vi "LJLogUD.vi"() -> ()   [LabVIEW 2020]
panel:
  in  "Save Current Config":bool
  out "Device Config File Name":string
  out "Actual Interval (ms)":i32
  in  "Graphing parameters":T1(tab)
  in  "Graph?":bool[](array[boolean])
  out "Scaled":dbl[](array[numeric]) format="%.6f"
  in  "Scaling Equation":string[](array[string])=["y=a", "y=b", "y=c", "y=d", "y=e", "y=f", "y=g", "y=h", "y=i", "y=j", "y=k", "y=l", "y=m", "y=n", "y=o", "y=p"]
  out "Voltage":dbl[](array[numeric]) format="%.6f"
  in  "Ranges":u16[](array[ring])=[0, 0, 0, 0, 0, 0, 0, 0, 0, 0, 0, 0, 0, 0, 0, 0] items=["LJ_rgBIP10V", "LJ_rgBIP5V", "LJ_rgUNI5V", "LJ_rgUNI2P5V", "LJ_rgUNI1P25V", "LJ_rgBIP1V", "LJ_rgUNIP625V", "LJ_rgBIPP1V", "LJ_rgBIPP01V"]
  in  "-Ch":string[](array[string])=["199", "199", "199", "199", "199", "199", "199", "199", "199", "199", "199", "199", "199", "199", "199", "199"]
  in  "+Ch":string[](array[string])=["1", "2", "3", "4", "5", "6", "7", "8", "9", "10", "11", "12", "13", "14", "15", "16"]
  out "Scaled 2":dbl[](array[numeric]) format="%.6f"
  in  "Graph? 2":bool[](array[boolean])
  in  "Ranges 2":u16[](array[ring])=[0, 0, 0, 0, 0, 0, 0, 0, 0, 0, 0, 0, 0, 0, 0, 0] items=["LJ_rgBIP10V", "LJ_rgBIP5V", "LJ_rgUNI5V", "LJ_rgUNI2P5V", "LJ_rgUNI1P25V", "LJ_rgBIP1V", "LJ_rgUNIP625V", "LJ_rgBIPP1V", "LJ_rgBIPP01V"]
  in  "Scaling Equation 2":string[](array[string])=["y=a2", "y=b2", "y=c2", "y=d2", "y=e2", "y=f2", "y=g2", "y=h2", "y=i2", "y=j2", "y=k2", "y=l2", "y=m2", "y=n2", "y=o2", "y=p2"]
  out "Voltage 2":dbl[](array[numeric]) format="%.6f"
  in  "-Ch 2":string[](array[string])=["199", "199", "199", "199", "199", "199", "199", "199", "199", "199", "199", "199", "199", "199", "199", "199"]
  in  "+Ch 2":string[](array[string])=["X3-AIN4", "X3-AIN5", "X3-AIN6", "X3-AIN7", "X3-AIN8", "X3-AIN9", "X3-AIN10", "X3-AIN11", "X3-AIN12", "X3-AIN13", "X3-DAC0", "X3-DAC1", "X3-FIO0", "X3-FIO1", "X3-FIO2", "X3-FIO3"]
  in  "Graph? 3":bool[](array[boolean])
  in  "Ranges 3":u16[](array[ring])=[0, 0, 0, 0, 0, 0, 0, 0, 0, 0, 0, 0, 0, 0, 0, 0] items=["LJ_rgBIP10V", "LJ_rgBIP5V", "LJ_rgUNI5V", "LJ_rgUNI2P5V", "LJ_rgUNI1P25V", "LJ_rgBIP1V", "LJ_rgUNIP625V", "LJ_rgBIPP1V", "LJ_rgBIPP01V"]
  out "Scaled 3":dbl[](array[numeric]) format="%.6f"
  in  "Scaling Equation 3":string[](array[string])=["y=a3", "y=b3", "y=c3", "y=d3", "y=e3", "y=f3", "y=g3", "y=h3", "y=i3", "y=j3", "y=k3", "y=l3", "y=m3", "y=n3", "y=o3", "y=p3"]
  out "Voltage 3":dbl[](array[numeric]) format="%.6f"
  in  "-Ch 3":string[](array[string])=["199", "199", "199", "199", "199", "199", "199", "199", "199", "199", "199", "199", "199", "199", "199", "199"]
  in  "+Ch 3":string[](array[string])=["X3-FIO4", "X3-FIO5", "X3-FIO6", "X3-FIO7", "X4-AIN0", "X4-AIN1", "X4-AIN2", "X4-AIN3", "X4-AIN4", "X4-AIN5", "X4-AIN6", "X4-AIN7", "X4-AIN8", "X4-AIN9", "X4-AIN10", "X4-AIN11"]
  in  "Graph? 4":bool[](array[boolean])
  in  "Ranges 4":u16[](array[ring])=[0, 0, 0, 0, 0, 0, 0, 0, 0, 0, 0, 0, 0, 0, 0, 0] items=["LJ_rgBIP10V", "LJ_rgBIP5V", "LJ_rgUNI5V", "LJ_rgUNI2P5V", "LJ_rgUNI1P25V", "LJ_rgBIP1V", "LJ_rgUNIP625V", "LJ_rgBIPP1V", "LJ_rgBIPP01V"]
  out "Scaled 4":dbl[](array[numeric]) format="%.6f"
  in  "Scaling Equation 4":string[](array[string])=["y=a4", "y=b4", "y=c4", "y=d4", "y=e4", "y=f4", "y=g4", "y=h4", "y=i4", "y=j4", "y=k4", "y=l4", "y=m4", "y=n4", "y=o4", "y=p4"]
  out "Voltage 4":dbl[](array[numeric]) format="%.6f"
  in  "-Ch 4":string[](array[string])=["199", "199", "199", "199", "199", "199", "199", "199", "199", "199", "199", "199", "199", "199", "199", "199"]
  in  "+Ch 4":string[](array[string])=["X4-AIN12", "X4-AIN13", "X4-DAC0", "X4-DAC1", "X4-FIO0", "X4-FIO1", "X4-FIO2", "X4-FIO3", "X4-FIO4", "X4-FIO5", "X4-FIO6", "X4-FIO7", "X5-AIN0", "X5-AIN1", "X5-AIN2", "X5-AIN3"]
  in  "Graph? 5":bool[](array[boolean])
  in  "Ranges 5":u16[](array[ring])=[0, 0, 0, 0, 0, 0, 0, 0, 0, 0, 0, 0, 0, 0, 0, 0] items=["LJ_rgBIP10V", "LJ_rgBIP5V", "LJ_rgUNI5V", "LJ_rgUNI2P5V", "LJ_rgUNI1P25V", "LJ_rgBIP1V", "LJ_rgUNIP625V", "LJ_rgBIPP1V", "LJ_rgBIPP01V"]
  out "Scaled 5":dbl[](array[numeric]) format="%.6f"
  in  "Scaling Equation 5":string[](array[string])=["y=a5", "y=b5", "y=c5", "y=d5", "y=e5", "y=f5", "y=g5", "y=h5", "y=i5", "y=j5", "y=k5", "y=l5", "y=m5", "y=n5", "y=o5", "y=p5"]
  out "Voltage 5":dbl[](array[numeric]) format="%.6f"
  in  "-Ch 5":string[](array[string])=["199", "199", "199", "199", "199", "199", "199", "199", "199", "199", "199", "199", "199", "199", "199", "199"]
  in  "+Ch 5":string[](array[string])=["X5-AIN4", "X5-AIN5", "X5-AIN6", "X5-AIN7", "X5-AIN8", "X5-AIN9", "X5-AIN10", "X5-AIN11", "X5-AIN12", "X5-AIN13", "X5-DAC0", "X5-DAC1", "X5-FIO0", "X5-FIO1", "X5-FIO2", "X5-FIO3"]
  in  "Graph? 6":bool[](array[boolean])
  in  "Ranges 6":u16[](array[ring])=[0, 0, 0, 0, 0, 0, 0, 0] items=["LJ_rgBIP10V", "LJ_rgBIP5V", "LJ_rgUNI5V", "LJ_rgUNI2P5V", "LJ_rgUNI1P25V", "LJ_rgBIP1V", "LJ_rgUNIP625V", "LJ_rgBIPP1V", "LJ_rgBIPP01V"]
  out "Scaled 6":dbl[](array[numeric]) format="%.6f"
  in  "Scaling Equation 6":string[](array[string])=["y=a6", "y=b6", "y=c6", "y=d6"]
  out "Voltage 6":dbl[](array[numeric]) format="%.6f"
  in  "-Ch 6":string[](array[string])=["199", "199", "199", "199"]
  in  "+Ch 6":string[](array[string])=["X5-FIO4", "X5-FIO5", "X5-FIO6", "X5-FIO7"]
  in  "Change Working Directory":bool
  in  "Max File Size (Bytes)":i32=1048576 min=1 max=2000000000
  out "Waveform Graph":cluster{dbl, dbl, dbl[][]}(graph)={0.0, 0.5, []}
  in  "# Scans On Graph":i32=1000 min=0
  out "Address":string
  out "Device Type":string
  in  "SettlingFactor":u8
  in  "Resolution":u8
  in  "exit":bool
  in  "# Channels":i32=4 min=1
  out "# Of Iterations":i32
  in  "Interval (ms)":u32=500
  out "Current Data File":path
  in  "Data File Prefix":string="data"
  in  "Write To File":bool
  out "Error Message":string="No Error"
  # "Page 1"
  # "Page 2"
  # "Page 3"
  # "Page 5"
  # "Page 6"
  # "Page 4"
  # "- \"a\" - \"p\" correspond to the raw Voltage value from \n  the 1st through 16th row of each page.\n- The scaled output value is \"y\".\n- If your equation has an error, the output will be\n   zero."
  # "0"
  # "1"
  # "2"
  # "3"
  # "4"
  # "5"
  # "6"
  # "7"
  # "8"
  # "9"
  # "10"
  # "11"
  # "12"
  # "13"
  # "14"
  # "15"
  # "+Ch"
  # "-Ch"
  # "Ranges"
  # "Voltage"
  # "Scaling Equation"
  # "Scaled"
  # "Graph?"
  # "16"
  # "17"
  # "18"
  # "19"
  # "20"
  # "21"
  # "22"
  # "23"
  # "24"
  # "25"
  # "26"
  # "27"
  # "28"
  # "29"
  # "30"
  # "31"
  # "+Ch"
  # "-Ch"
  # "Ranges"
  # "Voltage"
  # "Scaling Equation"
  # "Scaled"
  # "Graph?"
  # "32"
  # "33"
  # "34"
  # "35"
  # "36"
  # "37"
  # "38"
  # "39"
  # "40"
  # "41"
  # "42"
  # "43"
  # "44"
  # "45"
  # "46"
  # "47"
  # "+Ch"
  # "-Ch"
  # "Ranges"
  # "Voltage"
  # "Scaling Equation"
  # "Scaled"
  # "Graph?"
  # "48"
  # "49"
  # "50"
  # "51"
  # "52"
  # "53"
  # "54"
  # "55"
  # "56"
  # "57"
  # "58"
  # "59"
  # "60"
  # "61"
  # "62"
  # "63"
  # "+Ch"
  # "-Ch"
  # "Ranges"
  # "Voltage"
  # "Scaling Equation"
  # "Scaled"
  # "Graph?"
  # "64"
  # "65"
  # "66"
  # "67"
  # "68"
  # "69"
  # "70"
  # "71"
  # "72"
  # "73"
  # "74"
  # "75"
  # "76"
  # "77"
  # "78"
  # "79"
  # "+Ch"
  # "-Ch"
  # "Ranges"
  # "Voltage"
  # "Scaling Equation"
  # "Scaled"
  # "Graph?"
  # "80"
  # "81"
  # "82"
  # "83"
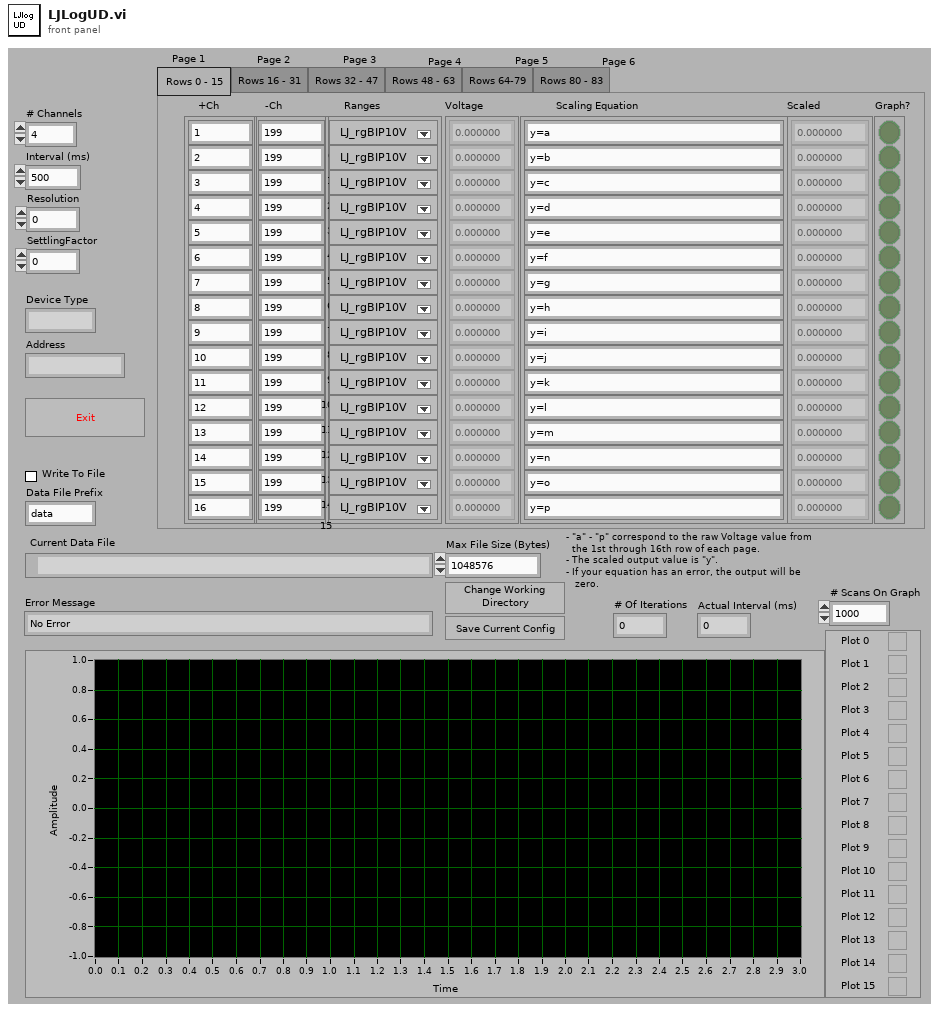
[diagram p1: front panel]
types:
  T1 = enum32{"Rows 0 - 15 ", "Rows 16 - 31", "Rows 32 - 47", "Rows 48 - 63", "Rows 64-79", "Rows 80 - 83"}
  T2 = cluster{"+Ch":string[], "-Ch":string[], "Ranges":u16[], "Scaling Equation":string[], "Graph?":bool[]}
  T3 = cluster{"# Channels":i32, "Channels Out":string[], "Channels Out":string[], u16[], string[]}
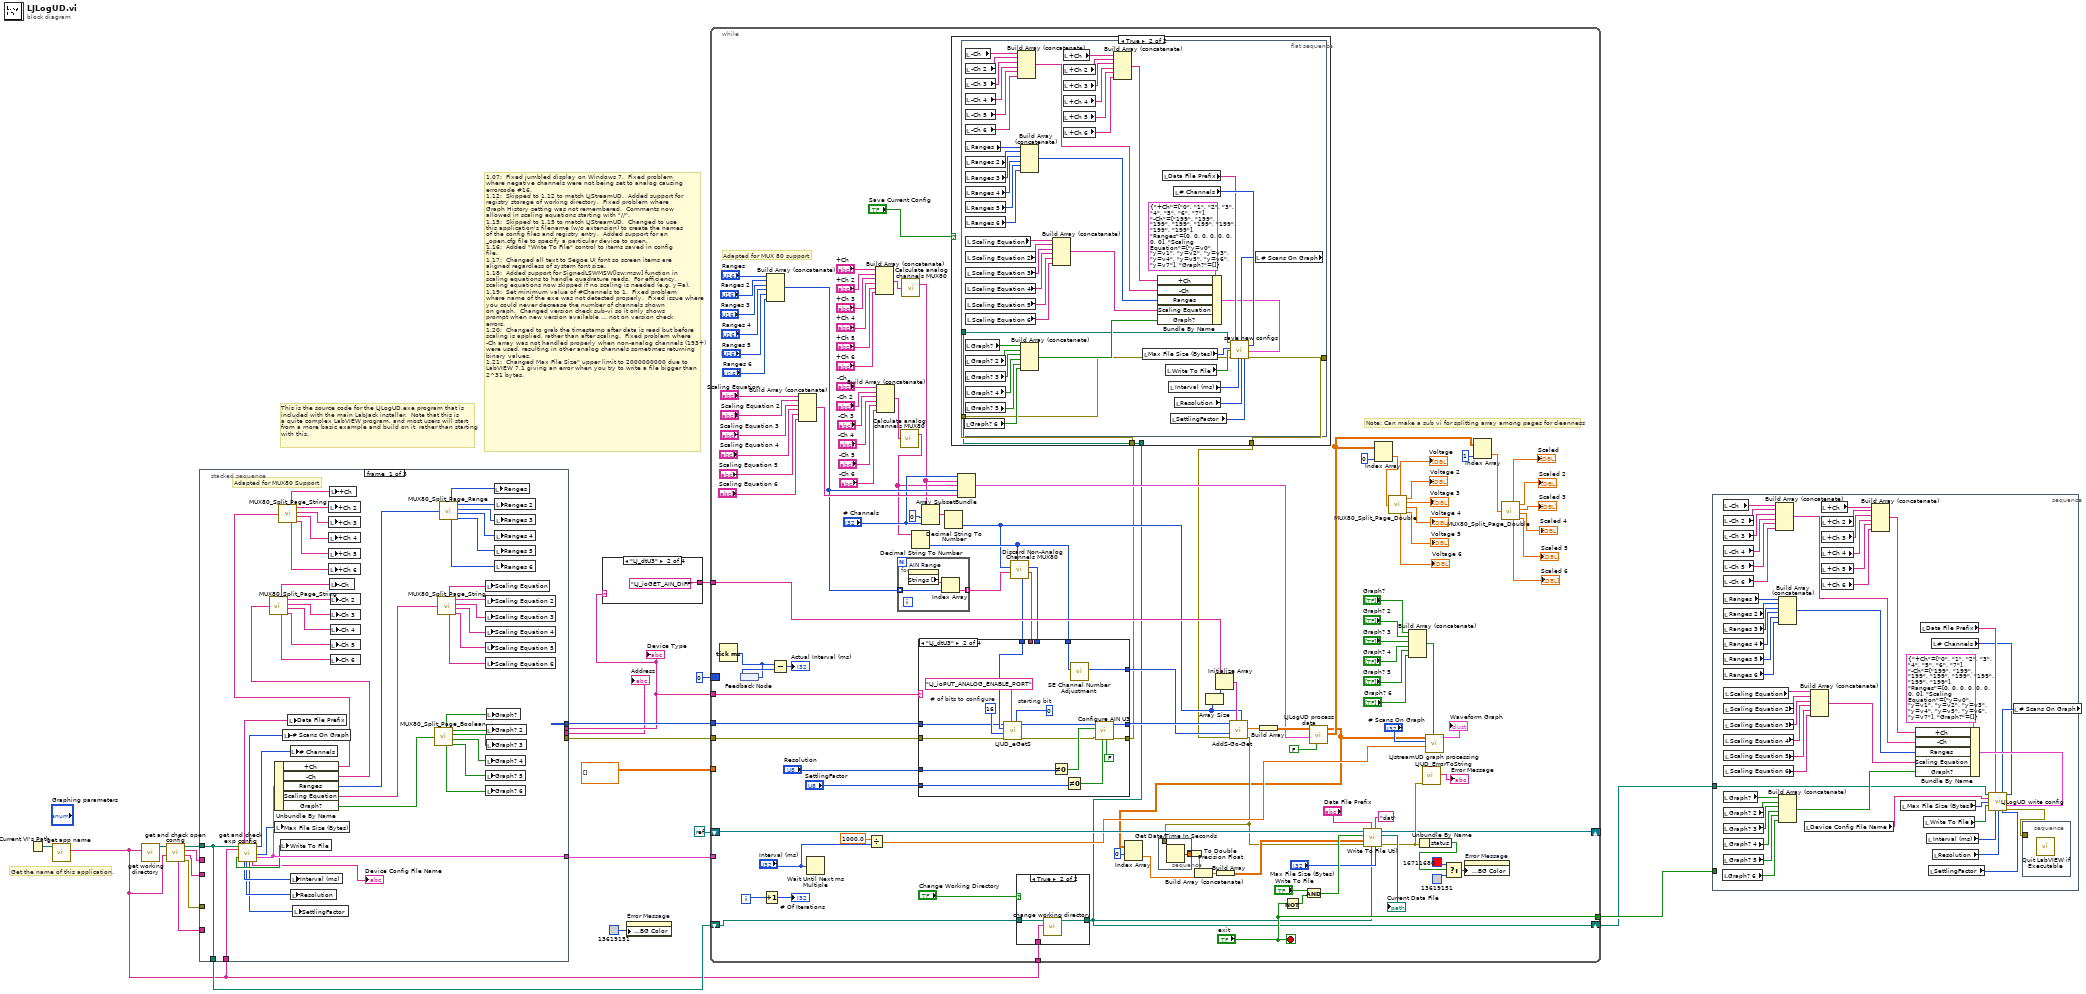
[diagram p0: block diagram]
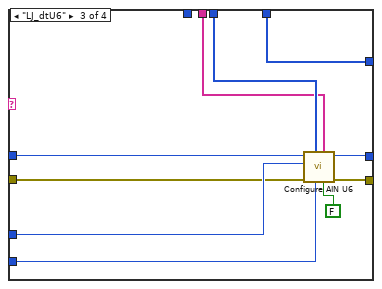
[diagram p5: hidden frame]
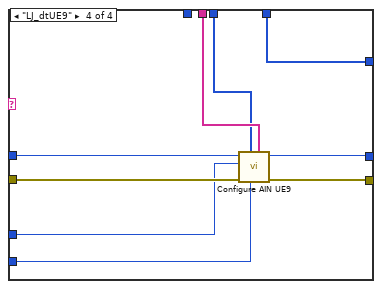
[diagram p6: hidden frame]
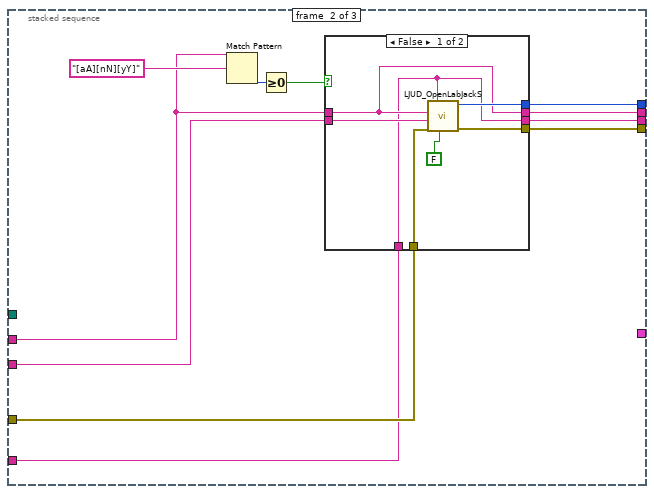
[diagram p7: hidden frame]
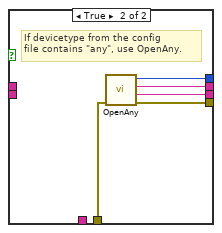
[diagram p8: hidden frame]
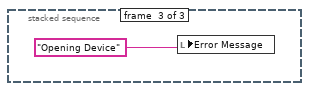
[diagram p9: hidden frame]
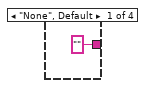
[diagram p10: hidden frame]
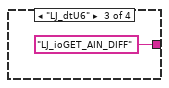
[diagram p11: hidden frame]
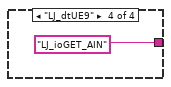
[diagram p12: hidden frame]
diagram:
  # "This is the source code for the LJLogUD.exe program that is\nincluded with the main LabJack installer.  Note that this is \na quite complex LabVIEW program, and most users will start\nfrom a more basic example and build on it, rather than starting\nwith this."
  # "Get the name of this application."
  # "1.07:  Fixed jumbled display on Windows 7.  Fixed problem\nwhere negative channels were not being set to analog causing\nerrorcode #16.\n1.12:  Skipped to 1.12 to match LJStreamUD.  Added support for\nregistry storage of working directory.  Fixed problem where\nGraph History setting was not remembered.  Comments now\nallowed in scaling equations starting with \"//\".\n1.15:  Skipped to 1.15 to match LJStreamUD.  Changed to use\nthis application's filename (w/o extension) to create the names\nof the config files and registry entry.  Added support for an\n_open.cfg file to specify a particular device to open.\n1.16:  Added \"Write To File\" control to items saved in config\nfile.\n1.17:  Changed all text to Segoe UI font so screen items are\naligned regardless of system font size.\n1.18:  Added support for SignedLSWMSW[lsw:msw] function in\nscaling equations to handle quadrature reads.  For efficiency,\nscaling equations now skipped if no scaling is needed (e.g. y=a).\n1.19:  Set minimum value of #Channels to 1.  Fixed problem\nwhere name of the exe was not detected properly.  Fixed issue where\nyou could never decrease the number of channels shown\non graph.  Changed version check sub-vi so it only shows\nprompt when new version available ... not on version check\nerrors.\n1.20:  Changed to grab the timestamp after data is read but before\nscaling is applied, rather than after scaling.  Fixed problem where\n-Ch array was not handled properly when non-analog channels (193+)\nwere used, resulting in other analog channels sometimes returning\nbinary values.\n1.21:  Changed Max File Size\" upper limit to 2000000000 due to\nLabVIEW 7.1 giving an error when you try to write a file bigger than\n2^31 bytes."
  n1 = Current VI's Path() -> (path=w10:path)
  n2 = call "get app name.vi"("Current VI's Path"=w10) -> ("App Name Without Extension"=w2:string)  [unwired: 4 in, 2 out]
  n3 = call "get working directory.vi"("Application Name"=w2) -> ("Working Directory"=w8:path)  [unwired: 9 in, 1 out]
  n4 = call "get and check open config.vi"("App Name"=w2, "Working Directory In"=w8) -> ("error out"=w6:errorcluster, "ConnectionType"=w4:string, "DeviceType"=w3:string, "Working Directory Out"=w7:path, "Identifier"=w5:string)  [unwired: 4 in, 1 out]
  n5 = stacked-sequence {
    tunnel: [w29 _ _] -> w18
    tunnel: [w26 _ _] -> w16
    tunnel: w2 -> [w33 _ _]
    tunnel: [_ w79 _] -> w14
    tunnel: [_ w78 _] -> w13
    tunnel: [_ w77 _] -> w12
    tunnel: [_ w76 _] -> w11
    tunnel: w7 -> [w26 _ _]
    tunnel: w6 -> [_ w72 _]
    tunnel: w5 -> [_ w71 _]
    tunnel: w4 -> [_ w70 _]
    tunnel: w3 -> [_ w69 _]
    frame #0 {
      # "Adapted for MUX80 Support"
      n6 = call "get and check exp config.vi"("Working Directory In"=w26, "App Name"=w33) -> ("Write To File"=w28:bool, "Data File Prefix"=w32:string, "Interval (ms)"=w27:u32, "Resolution"=w24:u8, "Graph History"=w31:i32, "SettlingFactor"=w23:u8, "Device Config File Name"=→"Device Config File Name":string, "# Channels"=w25:i32, "Max File Size (Bytes)"=w30:i32, "Channel Setup"=w29:T2)  [unwired: 6 in, 2 out]
      n7 = Unbundle By Name(w29) -> ("+Ch"=w56:string[], "-Ch"=w55:string[], "Ranges"=w47:u16[], "Scaling Equation"=w54:string[], "Graph?"=w40:bool[])
      n8 = call "MUX80_Split_Page_String.vi"("Array In"=w55) -> ("Page 1 out"=w62:string[], "Page 6 out"=w57:string[], "Page 2 out"=w61:string[], "Page 3 out"=w60:string[], "Page 4 out"=w59:string[], "Page 5 out"=w58:string[])
      n9 = local write "Max File Size (Bytes)"(w30) -> ()
      n10 = call "MUX80_Split_Page_String.vi"("Array In"=w56) -> ("Page 1 out"=w68:string[], "Page 6 out"=w63:string[], "Page 2 out"=w67:string[], "Page 3 out"=w66:string[], "Page 4 out"=w65:string[], "Page 5 out"=w64:string[])
      n11 = local write "Write To File"(w28) -> ()
      n12 = local write "# Scans On Graph"(w31) -> ()
      n13 = local write "Data File Prefix"(w32) -> ()
      n14 = local write "# Channels"(w25) -> ()
      n15 = local write "Interval (ms)"(w27) -> ()
      n16 = local write "Resolution"(w24) -> ()
      n17 = local write "SettlingFactor"(w23) -> ()
      n18 = local write "+Ch 2"(w67) -> ()
      n19 = local write "+Ch 3"(w66) -> ()
      n20 = local write "+Ch 4"(w65) -> ()
      n21 = local write "+Ch 5"(w64) -> ()
      n22 = local write "+Ch 6"(w63) -> ()
      n23 = local write "+Ch"(w68) -> ()
      n24 = local write "-Ch"(w62) -> ()
      n25 = local write "-Ch 2"(w61) -> ()
      n26 = local write "-Ch 3"(w60) -> ()
      n27 = local write "-Ch 4"(w59) -> ()
      n28 = local write "-Ch 5"(w58) -> ()
      n29 = local write "-Ch 6"(w57) -> ()
      n30 = call "MUX80_Split_Page_Boolean.vi"("Array In"=w40) -> ("Page 1 out"=w39:bool[], "Page 6 out"=w34:bool[], "Page 2 out"=w38:bool[], "Page 3 out"=w37:bool[], "Page 4 out"=w36:bool[], "Page 5 out"=w35:bool[])
      n31 = call "MUX80_Split_Page_String.vi"("Array In"=w54) -> ("Page 1 out"=w53:string[], "Page 6 out"=w48:string[], "Page 2 out"=w52:string[], "Page 3 out"=w51:string[], "Page 4 out"=w50:string[], "Page 5 out"=w49:string[])
      n32 = call "MUX80_Split_Page_Range.vi"("Array In"=w47) -> ("Page 1 out"=w46:u16[], "Page 6 out"=w41:u16[], "Page 2 out"=w45:u16[], "Page 3 out"=w44:u16[], "Page 4 out"=w43:u16[], "Page 5 out"=w42:u16[])
      n33 = local write "Scaling Equation"(w53) -> ()
      n34 = local write "Scaling Equation 2"(w52) -> ()
      n35 = local write "Scaling Equation 3"(w51) -> ()
      n36 = local write "Scaling Equation 4"(w50) -> ()
      n37 = local write "Scaling Equation 5"(w49) -> ()
      n38 = local write "Scaling Equation 6"(w48) -> ()
      n39 = local write "Graph? 4"(w36) -> ()
      n40 = local write "Graph? 5"(w35) -> ()
      n41 = local write "Graph? 6"(w34) -> ()
      n42 = local write "Graph?"(w39) -> ()
      n43 = local write "Graph? 2"(w38) -> ()
      n44 = local write "Graph? 3"(w37) -> ()
      n45 = local write "Ranges"(w46) -> ()
      n46 = local write "Ranges 2"(w45) -> ()
      n47 = local write "Ranges 3"(w44) -> ()
      n48 = local write "Ranges 4"(w43) -> ()
      n49 = local write "Ranges 5"(w42) -> ()
      n50 = local write "Ranges 6"(w41) -> ()
    }
    frame #1 {
      n51 = Match Pattern(string=w69, regular expression="[aA][nN][yY]") -> (offset past match=w75:i32)  [unwired: 1 in, 3 out]
      n52 = Greater Or Equal To 0?(x=w75) -> (x >= 0?=w73:bool)
      n53 = case shown="False" w73 {
        tunnel: [w86 w91] -> w79
        tunnel: [w82 w90] -> w78
        tunnel: [w80 w89] -> w77
        tunnel: [w85 w88] -> w76
        tunnel: w71 -> [w80 _]
        tunnel: w69 -> [w82 _]
        tunnel: w70 -> [w81 _]
        tunnel: w72 -> [w83 w87]
        frame False {
          n54 = call "LJUD_OpenLabJackS.vi"("FirstFound"=FALSE, "Address"=w80, "error in"=w83, "ConnectionType"=w81, "DeviceType"=w82) -> ("error out"=w85:errorcluster, "Handle"=w86:i32)  [unwired: 4 in, 1 out]
        }
        frame True {
          # "If devicetype from the config\nfile contains \"any\", use OpenAny."
          n55 = call "OpenAny.vi"("error in"=w87) -> ("error out"=w88:errorcluster, "Address Found"=w89:string, "Device Type Found"=w90:string, "Handle"=w91:i32)  [unwired: 7 in]
        }
      }
    }
    frame #2 {
      n56 = local write "Error Message"("Opening Device" ("Error Message")) -> ()
    }
  }
  "Device Type" <- w13
  "Address" <- w12
  n57 = case shown="\"LJ_dtU3\"" w13 {
    tunnel: ["" ("IOType") "LJ_ioGET_AIN_DIFF" ("IOType") "LJ_ioGET_AIN_DIFF" ("IOType") "LJ_ioGET_AIN" ("IOType")] -> w20
    frame "None", Default {
    }
    frame "LJ_dtU3" {
    }
    frame "LJ_dtU6" {
    }
    frame "LJ_dtUE9" {
    }
  }
  n58 = property on="Error Message" class="Str"("Text.Text Colors:BG Color"=u32 13619151) -> ()  [unwired: 2 in, 2 out]
  n59 = while {
    shift-left: w16 -> [w99]
    shift-right: [w98] -> w15
    tunnel: w2 -> [w170]
    tunnel: dbl[][] [] ("Waveform Chart") -> [_]
    tunnel: w20 -> [w188]
    tunnel: w11 -> [w189]
    tunnel: w13 -> [w197]
    tunnel: w14 -> [w196]
    shift-left: refnum<k0> refnum -> [w200]
    shift-right: [w105] -> _
    tunnel: w18 -> [_]
    tunnel: ["exit"] -> w17
    border: 0 -> [_]
    i -> [w206]
    stop <- "exit" stop-if-true
    # "Adapted for MUX 80 support"
    # "Note: Can make a sub vi for splitting array among pages for cleanness"
    n60 = Tick Count (ms)() -> (millisecond timer value=w103:u32)
    n61 = feedback-in #1(w103) -> ()
    n62 = feedback #1() -> (w104:u32)
    n63 = Increment(x=w206) -> (x+1=→"# Of Iterations":i32)
    n64 = Build Array (concatenate)("Ranges", "Ranges 2", "Ranges 3", "Ranges 4", "Ranges 5", "Ranges 6") -> (w149:u16[])
    n65 = Subtract(x=w103, y=w104) -> (x-y=→"Actual Interval (ms)":u32)
    n66 = Build Array (concatenate)("Scaling Equation", "Scaling Equation 2", "Scaling Equation 3", "Scaling Equation 4", "Scaling Equation 5", "Scaling Equation 6") -> (w155:string[])
    n67 = Wait Until Next ms Multiple(millisecond multiple="Interval (ms)") -> ()  [unwired: 1 out]
    n68 = Divide(x=1000.0, y="Interval (ms)") -> (x/y=w179:dbl)
    n69 = Build Array (concatenate)("+Ch", "+Ch 2", "+Ch 3", "+Ch 4", "+Ch 5", "+Ch 6") -> (w109:string[])
    n70 = Build Array (concatenate)("-Ch", "-Ch 2", "-Ch 3", "-Ch 4", "-Ch 5", "-Ch 6") -> (w107:string[])
    n71 = for {
      tunnel: w149 -> [w312] mode=indexing
      tunnel: [w311] -> w110 mode=indexing
      n72 = property on="AIN Range" class="Ring (strict)"() -> ("Strings []"=w313:string[])  [unwired: 2 in, 2 out]
      n73 = Index Array(array=w313, index=w312) -> (element=w311:string)
    }
    n74 = call "Calculate analog channels MUX80.vi"("Channels In"=w107) -> ("Channels Out"=w106:string[])  [unwired: 1 out]
    n75 = call "Calculate analog channels MUX80.vi"("Channels In"=w109) -> ("Channels Out"=w108:string[])  [unwired: 1 out]
    n76 = Decimal String To Number(string=w106) -> (number=w115:i32[])  [unwired: 2 in, 1 out]
    n77 = Array Subset(array=w108, index=0 ("Array Index"), length="# Channels") -> (w207:string[])
    n78 = Decimal String To Number(string=w207) -> (number=w114:i32[])  [unwired: 2 in, 1 out]
    n79 = Bundle("# Channels"="# Channels", "Channels Out"=w108, "Channels Out"=w106, w149, w155) -> (w117:T3)  [unwired: 1 in]
    n80 = call "Discard Non-Analog Channels MUX80.vi"("Channels In (-)"=w115, "Ranges In"=w110, "Channels In"=w114) -> ("Ranges Out"=w111:string[], "Channels Out"=w112:i32[], "FIO/EIO Analog Enable"=w113:i32)  [unwired: 5 in, 1 out]
    n81 = case shown="\"LJ_dtU3\"" w197 {
      tunnel: w113 -> [_ w280 _ _]
      tunnel: w189 -> [w274 w279 w293 w309]
      tunnel: w196 -> [w273 w278 w294 w310]
      tunnel: [w274 w286 w300 w306] -> w101
      tunnel: [w273 w287 w301 w307] -> w192
      tunnel: w111 -> [_ _ w298 w308]
      tunnel: w112 -> [_ _ w299 w302]
      tunnel: "Resolution" -> [_ w291 w297 w305]
      tunnel: "SettlingFactor" -> [_ w289 w296 w304]
      tunnel: [w272 w285 w292 w303] -> w191
      tunnel: w115 -> [w272 w275 w292 w303]
      frame "None", Default {
      }
      frame "LJ_dtU3" {
        w282 = 0  # starting bit
        w283 = 16  # # of bits to configure
        n82 = call "LJUD_eGetS.vi"("Channel"=w282, "IOType"="LJ_ioPUT_ANALOG_ENABLE_PORT" ("Channel"), "error in"=w279, "x1"=w283, "Value Write"=w280, "Handle In"=w278) -> ("error out"=w277:errorcluster, "Handle Out"=w276:i32)  [unwired: 3 in, 1 out]
        n83 = Not Equal To 0?(x=w291) -> (x != 0?=w290:bool)
        n84 = Not Equal To 0?(x=w289) -> (x != 0?=w288:bool)
        n85 = call "SE Channel Number Adjustment.vi"("Channels In"=w275) -> ("Channels Out"=w285:i32[])  [unwired: 10 in]
        n86 = call "Configure AIN U3.vi"("Binary"=FALSE ("Enable DAC1"), "longSettling"=w288, "error in"=w277, "quickSample"=w290, "Handle In"=w276) -> ("error out"=w286:errorcluster, "Handle Out"=w287:i32)  [unwired: 5 in]
      }
      frame "LJ_dtU6" {
        n87 = call "Configure AIN U6.vi"("Binary"=FALSE ("Enable Counter0"), "Ranges"=w298, "SettlingFactor"=w296, "Positive Channels"=w299, "error in"=w293, "Resolution"=w297, "Handle In"=w294) -> ("error out"=w300:errorcluster, "Handle Out"=w301:i32)  [unwired: 3 in]
      }
      frame "LJ_dtUE9" {
        n88 = call "Configure AIN UE9.vi"("Ranges"=w308, "SettlingFactor"=w304, "Channels"=w302, "error in"=w309, "Resolution"=w305, "Handle In"=w310) -> ("error out"=w306:errorcluster, "Handle Out"=w307:i32)  [unwired: 4 in]
      }
    }
    n89 = case shown="True" "Change Working Directory" {
      tunnel: w170 -> [_ w269]
      tunnel: w99 -> [w266 w268]
      tunnel: [w266 w267] -> w98
      frame False {
      }
      frame True {
        n90 = call "change working directory.vi"("Application Name"=w269, "Working Directory In"=w268) -> ("Working Directory Out"=w267:path)  [unwired: 9 in]
      }
    }
    n91 = case shown="True" "Save Current Config" {
      tunnel: w101 -> [w214 w217]
      tunnel: w98 -> [_ w216]
      tunnel: [w214 w215] -> w100
      frame False {
      }
      frame True {
        n92 = flat-sequence {
          tunnel: w217 -> [w221]
          tunnel: w216 -> [w220]
          tunnel: [w219] -> w215
          frame #0 {
            n93 = local read "Graph? 6"() -> (w253:bool[])
            n94 = local read "-Ch"() -> (w218:string[])
            n95 = local read "-Ch 2"() -> (w231:string[])
            n96 = local read "-Ch 3"() -> (w232:string[])
            n97 = local read "-Ch 4"() -> (w233:string[])
            n98 = local read "-Ch 5"() -> (w234:string[])
            n99 = local read "-Ch 6"() -> (w235:string[])
            n100 = local read "Ranges"() -> (w236:u16[])
            n101 = local read "Ranges 2"() -> (w237:u16[])
            n102 = local read "Ranges 3"() -> (w238:u16[])
            n103 = local read "Ranges 4"() -> (w239:u16[])
            n104 = local read "Ranges 5"() -> (w240:u16[])
            n105 = local read "Ranges 6"() -> (w241:u16[])
            n106 = local read "Graph?"() -> (w248:bool[])
            n107 = local read "Graph? 2"() -> (w249:bool[])
            n108 = local read "Graph? 3"() -> (w250:bool[])
            n109 = local read "Graph? 4"() -> (w251:bool[])
            n110 = local read "Graph? 5"() -> (w252:bool[])
            n111 = local read "Scaling Equation"() -> (w242:string[])
            n112 = local read "Scaling Equation 2"() -> (w243:string[])
            n113 = local read "Scaling Equation 3"() -> (w244:string[])
            n114 = local read "Scaling Equation 4"() -> (w245:string[])
            n115 = local read "Scaling Equation 5"() -> (w246:string[])
            n116 = local read "Scaling Equation 6"() -> (w247:string[])
            n117 = Build Array (concatenate)(w218, w231, w232, w233, w234, w235) -> (w255:string[])
            n118 = Build Array (concatenate)(w236, w237, w238, w239, w240, w241) -> (w256:u16[])
            n119 = Build Array (concatenate)(w248, w249, w250, w251, w252, w253) -> (w258:bool[])
            n120 = Build Array (concatenate)(w242, w243, w244, w245, w246, w247) -> (w257:string[])
            n121 = local read "+Ch"() -> (w225:string[])
            n122 = local read "+Ch 2"() -> (w226:string[])
            n123 = local read "+Ch 3"() -> (w227:string[])
            n124 = local read "+Ch 4"() -> (w228:string[])
            n125 = local read "+Ch 5"() -> (w229:string[])
            n126 = local read "+Ch 6"() -> (w230:string[])
            n127 = Build Array (concatenate)(w225, w226, w227, w228, w229, w230) -> (w254:string[])
            n128 = local read "Max File Size (Bytes)"() -> (w264:i32)
            n129 = Bundle By Name(cluster=T2 {"+Ch"=["0", "1", "2", "3", "4", "5", "6", "7"], "-Ch"=["199", "199", "199", "199", "199", "199", "199", "199"], "Ranges"=[0, 0, 0, 0, 0, 0, 0, 0], "Scaling Equation"=["y=v0", "y=v1", "y=v2", "y=v3", "y=v4", "y=v5", "y=v6", "y=v7"], "Graph?"=[]} ("Channel Setup"), "+Ch"=w254, "-Ch"=w255, "Ranges"=w256, "Scaling Equation"=w257, "Graph?"=w258) -> (w223:T2)
            n130 = local read "Data File Prefix"() -> (w260:string)
            n131 = local read "Write To File"() -> (w262:bool)
            n132 = local read "Interval (ms)"() -> (w259:u32)
            n133 = local read "SettlingFactor"() -> (w222:u8)
            n134 = local read "# Channels"() -> (w265:i32)
            n135 = local read "Resolution"() -> (w263:u8)
            n136 = local read "# Scans On Graph"() -> (w261:i32)
            n137 = call "save new configs.vi"("Working Directory"=w220, "Max File Size (Bytes)"=w264, "Write To File"=w262, "error in"=w221, "Data File Prefix"=w260, "Interval (ms)"=w259, "Graph History"=w261, "Resolution"=w263, "# Channels"=w265, "SettlingFactor"=w222, "Channel Setup"=w223) -> ("error out"=w219:errorcluster)  [unwired: 7 in, 1 out]
          }
        }
      }
    }
    n138 = Array Size(array=w114) -> (size(s)=w199:i32)
    n139 = Initialize Array(w188, w199) -> (w198:string[])
    n140 = call "AddS-Go-Get.vi"("Channels"=w114, "IOTypes"=w198, "error in"=w100, "x1"=w191, "Handle In"=w192) -> ("error out"=w169:errorcluster, "Values Read"=w193:dbl[])  [unwired: 4 in, 1 out]
    n141 = stacked-sequence {
      tunnel: [w271] -> w187
      tunnel: w169 -> [_]
      frame #0 {
        n142 = Get Date/Time In Seconds() -> (seconds since 1Jan1904=w270:timestamp)
        n143 = To Double Precision Float(number=w270) -> (double precision float=w271:dbl)
      }
    }
    n144 = Build Array(w193) -> (w118:dbl[][])
    n145 = Not(x="exit") -> (.not. x?=w209:bool)
    n146 = And(x="Write To File", y=w209) -> (x .and. y?=w201:bool)
    n147 = call "LJLogUD process data.vi"("Disable Scaling"=FALSE, "Channel Config"=w117, "Voltages"=w118) -> ("Volts,Scaled Averages"=w120:dbl[][], "Scaled Data"=w119:dbl[][])  [unwired: 7 in]
    n148 = Index Array(array=w119, index (row)=0 ("Index (row)")) -> (element=w184:dbl[])  [unwired: 1 in]
    n149 = Build Array (concatenate)(w187, w184) -> (w186:dbl[])
    n150 = Build Array(w186) -> (w183:dbl[][])
    n151 = call "Write To File Util.vi"("Maximum File Size (Bytes)"="Max File Size (Bytes)", "Data File Extension"="dat", "Working Directory"=w98, "Data File Prefix"="Data File Prefix", "error in"=w169, "Data"=w183, "Write To File"=w201, "File Refnum In"=w200) -> ("error out"=w176:errorcluster, "Current Data File"=→"Current Data File":path, "File Refnum Out"=w105:refnum<file>)  [unwired: 1 in]
    n152 = Index Array(array=w120, index (col)=0 ("Disabled Index (col)")) -> (element=w121:dbl[])  [unwired: 1 in]
    n153 = call "MUX80_Split_Page_Double.vi"("Array In"=w121) -> ("Page 1 out"=→"Voltage":dbl[], "Page 6 out"=→"Voltage 6":dbl[], "Page 2 out"=→"Voltage 2":dbl[], "Page 3 out"=→"Voltage 3":dbl[], "Page 4 out"=→"Voltage 4":dbl[], "Page 5 out"=→"Voltage 5":dbl[])
    n154 = Build Array (concatenate)("Graph?", "Graph? 2", "Graph? 3", "Graph? 4", "Graph? 5", "Graph? 6") -> (w162:bool[])
    n155 = Unbundle By Name(w176) -> ("status"=w175:bool)
    n156 = call "LJUD_ErrorToString.vi"("error in"=w176) -> ("String"=→"Error Message":string)  [unwired: 10 in]
    n157 = call "LJstreamUD graph processing.vi"("Graph?"=w162, "Scan Rate"=w179, "Graph History (# scans)"="# Scans On Graph", "Scaled Data"=w119) -> ("Graph Data"=→"Waveform Graph":cluster{dbl, dbl, dbl[][]})  [unwired: 7 in]
    n158 = Select(t=u32 16711680, s=w175, f=u32 13619151) -> (s? t:f=w174:u32)
    n159 = property on="Error Message" class="Str"("Text.Text Colors:BG Color"=w174) -> ()  [unwired: 2 in, 2 out]
    n160 = Index Array(array=w120, index (col)=1 ("Disabled Index (col)")) -> (element=w132:dbl[])  [unwired: 1 in]
    n161 = call "MUX80_Split_Page_Double.vi"("Array In"=w132) -> ("Page 1 out"=→"Scaled":dbl[], "Page 6 out"=→"Scaled 6":dbl[], "Page 2 out"=→"Scaled 2":dbl[], "Page 3 out"=→"Scaled 3":dbl[], "Page 4 out"=→"Scaled 4":dbl[], "Page 5 out"=→"Scaled 5":dbl[])
  }
  n162 = stacked-sequence {
    tunnel: w15 -> [w316]
    tunnel: w17 -> [_]
    frame #0 {
      n163 = local read "Graph? 6"() -> (w331:bool[])
      n164 = local read "-Ch"() -> (w354:string[])
      n165 = local read "-Ch 2"() -> (w353:string[])
      n166 = local read "-Ch 3"() -> (w352:string[])
      n167 = local read "-Ch 4"() -> (w351:string[])
      n168 = local read "-Ch 5"() -> (w350:string[])
      n169 = local read "-Ch 6"() -> (w349:string[])
      n170 = local read "Ranges"() -> (w348:u16[])
      n171 = local read "Ranges 2"() -> (w347:u16[])
      n172 = local read "Ranges 3"() -> (w346:u16[])
      n173 = local read "Ranges 4"() -> (w345:u16[])
      n174 = local read "Ranges 5"() -> (w344:u16[])
      n175 = local read "Ranges 6"() -> (w343:u16[])
      n176 = local read "Graph?"() -> (w336:bool[])
      n177 = local read "Graph? 2"() -> (w335:bool[])
      n178 = local read "Graph? 3"() -> (w334:bool[])
      n179 = local read "Graph? 4"() -> (w333:bool[])
      n180 = local read "Graph? 5"() -> (w332:bool[])
      n181 = local read "Scaling Equation"() -> (w342:string[])
      n182 = local read "Scaling Equation 2"() -> (w341:string[])
      n183 = local read "Scaling Equation 3"() -> (w340:string[])
      n184 = local read "Scaling Equation 4"() -> (w339:string[])
      n185 = local read "Scaling Equation 5"() -> (w338:string[])
      n186 = local read "Scaling Equation 6"() -> (w337:string[])
      n187 = Build Array (concatenate)(w354, w353, w352, w351, w350, w349) -> (w329:string[])
      n188 = Build Array (concatenate)(w348, w347, w346, w345, w344, w343) -> (w328:u16[])
      n189 = Build Array (concatenate)(w336, w335, w334, w333, w332, w331) -> (w326:bool[])
      n190 = local read "Device Config File Name"() -> (w314:string)
      n191 = Build Array (concatenate)(w342, w341, w340, w339, w338, w337) -> (w327:string[])
      n192 = local read "+Ch"() -> (w360:string[])
      n193 = local read "+Ch 2"() -> (w359:string[])
      n194 = local read "+Ch 3"() -> (w358:string[])
      n195 = local read "+Ch 4"() -> (w357:string[])
      n196 = local read "+Ch 5"() -> (w356:string[])
      n197 = local read "+Ch 6"() -> (w355:string[])
      n198 = Build Array (concatenate)(w360, w359, w358, w357, w356, w355) -> (w330:string[])
      n199 = local read "Max File Size (Bytes)"() -> (w317:i32)
      n200 = Bundle By Name(cluster=T2 {"+Ch"=["0", "1", "2", "3", "4", "5", "6", "7"], "-Ch"=["199", "199", "199", "199", "199", "199", "199", "199"], "Ranges"=[0, 0, 0, 0, 0, 0, 0, 0], "Scaling Equation"=["y=v0", "y=v1", "y=v2", "y=v3", "y=v4", "y=v5", "y=v6", "y=v7"], "Graph?"=[]} ("Channel Setup"), "+Ch"=w330, "-Ch"=w329, "Ranges"=w328, "Scaling Equation"=w327, "Graph?"=w326) -> (w325:T2)
      n201 = local read "Data File Prefix"() -> (w321:string)
      n202 = local read "Write To File"() -> (w319:bool)
      n203 = local read "Interval (ms)"() -> (w322:u32)
      n204 = local read "SettlingFactor"() -> (w323:u8)
      n205 = local read "# Channels"() -> (w315:i32)
      n206 = local read "Resolution"() -> (w318:u8)
      n207 = local read "# Scans On Graph"() -> (w320:i32)
      n208 = call "LJLogUD write config.vi"("Working Directory"=w316, "Data File Prefix"=w321, "Graph History"=w320, "# Channels"=w315, "filename"=w314, "Max File Size (Bytes)"=w317, "Write To File"=w319, "Channel Setup"=w325, "Interval (ms)"=w322, "Resolution"=w318, "SettlingFactor"=w323) -> ("error out"=w324:errorcluster)  [unwired: 4 in]
      n209 = stacked-sequence {
        tunnel: w324 -> [_]
        frame #0 {
          n210 = call "Quit LabVIEW if Executable.vi"() -> ()  [unwired: 1 in]
        }
      }
    }
  }
